vi "MoveToArena.vi"   [LabVIEW 2016, in "Moving Motor.lvrbt"]
uses:
  Moving Motor.lvrbt
  <vilib>/NXT/Hardware/Plugins/Tetrix DC Motor/TetrixDCMotorAddress.ctl
  <vilib>/NXT/Block Support/NXT_InputPort.ctl
  <vilib>/NXT/NXTIO Xnodes/NXTIONodeSubVIs/TETRIX IO Move DC Motors.vi
  <vilib>/NXT/Dual Mode Library/Waits/Wait_Num(msec).vi
  <vilib>/NXT/NXTIO Xnodes/NXTIONodeSubVIs/TETRIX IO Stop DC Motors.vi
  <vilib>/NXT/Dual Mode Library/Sensors/EV3_Color_Color.vi
  <vilib>/NXT/Subs/LVHSConnector.ctl
  <vilib>/NXT/NXTIO Xnodes/AddressXNode/NXTIOAddress.xnode
  <vilib>/NXT/NXTIO Xnodes/NXTIOXNode/NXTIO.xnode
  <vilib>/NXT/LegoClasses/BrickReference/BrickReference.lvclass
types:
  T1 = typedef "TetrixDCMotorAddress.ctl" = i32
  T2 = typedef "LVHSConnector.ctl" = refnum<class "BrickReference.lvclass">
  T3 = cluster{"TetrixDCMotor":T1, "TetrixDCMotor 2":T1}
  T4 = typedef "NXT_InputPort.ctl" = u32
  T5 = typedef "ColorSensorColors.ctl" = enum16{"No Color", "Black", "Blue", "Green", "Yellow", "Red", "White", "Brown"}
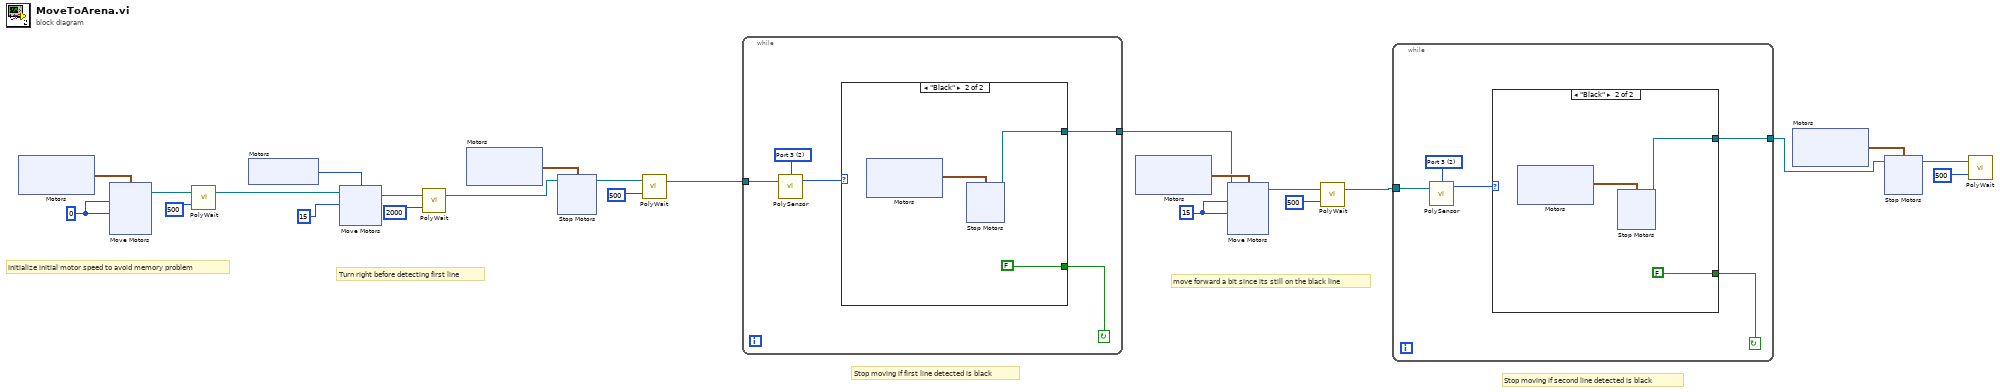
[diagram p0: block diagram]
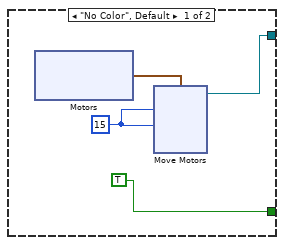
[diagram p2: hidden frame]
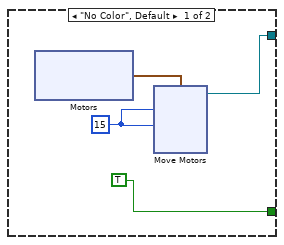
[diagram p3: hidden frame]
diagram:
  w10 = 15
  w23 = 0
  # "move forward a bit since its still on the black line"
  # "Stop moving if second line detected is black"
  # "Turn right before detecting first line"
  # "Stop moving if first line detected is black"
  # "Initialize initial motor speed to avoid memory problem"
  n1 = xnode "Motors"() -> ("Motor"=w24:cluster{"TetrixDCMotor":T1, "TetrixDCMotor":T1})
  n2 = xnode "Move Motors"("Power/Speed 2"=w23, "Power/Speed 1"=w23, "Motors"=w24) -> ("NXT/EV3"=w21:T2)  [unwired: 1 in]
  n3 = call-poly <vilib>:"PolyWait.vi"("Time (100 msec)"=500, "NXT/EV3"=w21) -> ("NXT/EV3"=w16:T2)  [unwired: 2 in]
  n4 = xnode "Motors"() -> ("Motor"=w20:T1)
  n5 = xnode "Move Motors"("Power/Speed 1"=15, "Motors"=w20, "NXT/EV3"=w16) -> ("NXT/EV3"=w17:T2)
  n6 = call-poly <vilib>:"PolyWait.vi"("Time (100 msec)"=2000, "NXT/EV3"=w17) -> ("NXT/EV3"=w14:T2)  [unwired: 2 in]
  n7 = xnode "Motors"() -> ("Motor"=w15:cluster{"TetrixDCMotor":T1, "TetrixDCMotor":T1})
  n8 = xnode "Stop Motors"("Motors"=w15, "NXT/EV3"=w14) -> ("NXT/EV3"=w13:T2)
  n9 = call-poly <vilib>:"PolyWait.vi"("Time (100 msec)"=500, "NXT/EV3"=w13) -> ("NXT/EV3"=w12:T2)  [unwired: 2 in]
  n10 = while {
    tunnel: w12 -> [w28]
    tunnel: [w25] -> w8
    stop <- w26 continue-if-true
    w29 = T4 2 items=["Port 1", "Port 2", "Port 3", "Port 4"] ("Port (Port 1)")
    n11 = call-poly <vilib>:"PolySensor.vi"("NXT/EV3"=w28, "Port (Port 1)"=w29) -> ("Detected Color"=w27:T5)  [unwired: 1 in, 1 out]
    n12 = case shown="\"Black\"" w27 {
      tunnel: [TRUE FALSE] -> w26
      tunnel: [w30 w43] -> w25
      frame "No Color", Default {
        w33 = 15
        n13 = xnode "Motors"() -> ("Motor"=w32:cluster{"TetrixDCMotor":T1, "TetrixDCMotor":T1})
        n14 = xnode "Move Motors"("Power/Speed 2"=w33, "Power/Speed 1"=w33, "Motors"=w32) -> ("NXT/EV3"=w30:T2)  [unwired: 1 in]
      }
      frame "Black" {
        n15 = xnode "Motors"() -> ("Motor"=w45:cluster{"TetrixDCMotor":T1, "TetrixDCMotor":T1})
        n16 = xnode "Stop Motors"("Motors"=w45) -> ("NXT/EV3"=w43:T2)  [unwired: 1 in]
      }
    }
  }
  n17 = xnode "Motors"() -> ("Motor"=w9:cluster{"TetrixDCMotor":T1, "TetrixDCMotor":T1})
  n18 = xnode "Move Motors"("Power/Speed 2"=w10, "Power/Speed 1"=w10, "Motors"=w9, "NXT/EV3"=w8) -> ("NXT/EV3"=w6:T2)
  n19 = call-poly <vilib>:"PolyWait.vi"("Time (100 msec)"=500, "NXT/EV3"=w6) -> ("NXT/EV3"=w5:T2)  [unwired: 2 in]
  n20 = while {
    tunnel: w5 -> [w55]
    tunnel: [w52] -> w1
    stop <- w53 continue-if-true
    w56 = T4 2 items=["Port 1", "Port 2", "Port 3", "Port 4"] ("Port (Port 1)")
    n21 = call-poly <vilib>:"PolySensor.vi"("NXT/EV3"=w55, "Port (Port 1)"=w56) -> ("Detected Color"=w54:T5)  [unwired: 1 in, 1 out]
    n22 = case shown="\"Black\"" w54 {
      tunnel: [TRUE FALSE] -> w53
      tunnel: [w57 w70] -> w52
      frame "No Color", Default {
        w60 = 15
        n23 = xnode "Motors"() -> ("Motor"=w59:cluster{"TetrixDCMotor":T1, "TetrixDCMotor":T1})
        n24 = xnode "Move Motors"("Power/Speed 2"=w60, "Power/Speed 1"=w60, "Motors"=w59) -> ("NXT/EV3"=w57:T2)  [unwired: 1 in]
      }
      frame "Black" {
        n25 = xnode "Motors"() -> ("Motor"=w72:cluster{"TetrixDCMotor":T1, "TetrixDCMotor":T1})
        n26 = xnode "Stop Motors"("Motors"=w72) -> ("NXT/EV3"=w70:T2)  [unwired: 1 in]
      }
    }
  }
  n27 = xnode "Motors"() -> ("Motor"=w4:cluster{"TetrixDCMotor":T1, "TetrixDCMotor":T1})
  n28 = xnode "Stop Motors"("Motors"=w4, "NXT/EV3"=w1) -> ("NXT/EV3"=w3:T2)
  n29 = call-poly <vilib>:"PolyWait.vi"("Time (100 msec)"=500, "NXT/EV3"=w3) -> ()  [unwired: 2 in, 1 out]
